vi "Convert Input Condition to Initial State.vi"(1 "Input Conditions":T2) -> (0 "Initial State":T1)   [LabVIEW 2022 SP3]
doc: "See \"Design Spreadsheet.xlsx\" for details"
uses:
  Input Conditions (cluster).ctl
  DFS Output (cluster).ctl
  Initial State (enum).ctl
panel:
  # "Development\nControls or indicators that are useful for development or testing, but which are not outputs of the VI."
  # "Input\nInputs to the VI"
  # "Output\nOutputs of the VI"
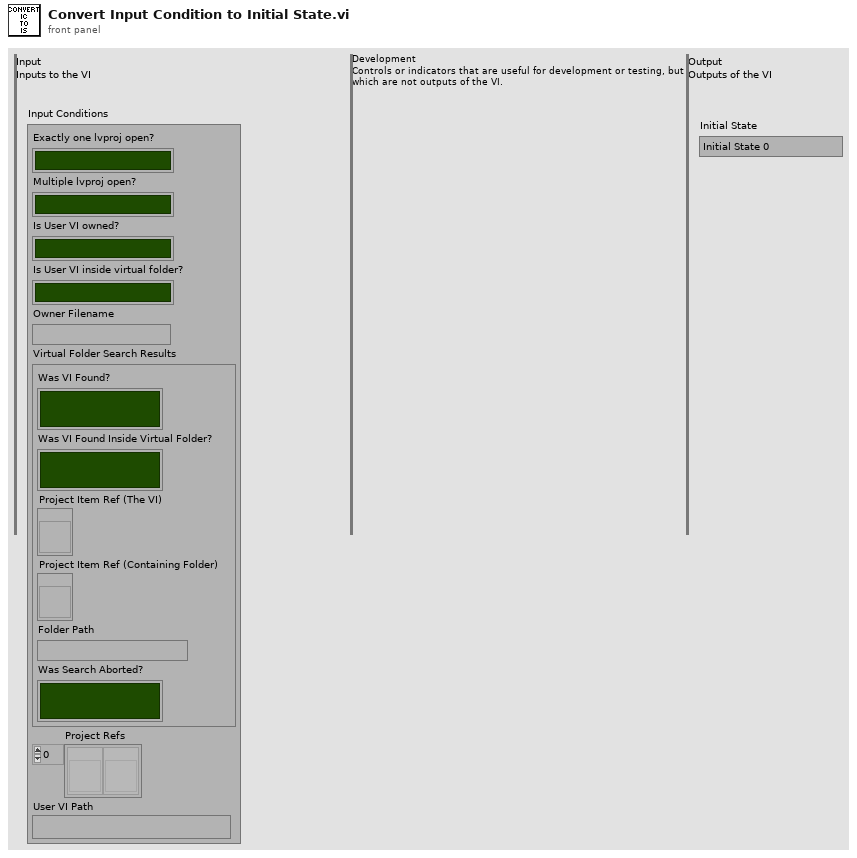
[diagram p1: front panel]
types:
  T1 = typedef "Initial State (enum).ctl" = enum16{"Initial State 0", "Initial State 1", "Initial State 2", "Initial State 3", "Initial State 4", "Initial State 5", "Initial State 6", "Initial State 7", "Initial State 8", "Initial State 9", "Initial State 10", "Initial State 11", "Initial State 12", "Initial State 13", "Initial State 14", "Initial State 15"}
  T2 = typedef "Input Conditions (cluster).ctl" = cluster{"Exactly one lvproj open?":bool, "Multiple lvproj open?":bool, "Is User VI owned?":bool, "Is User VI inside virtual folder?":bool, "Owner Filename":string, "Virtual Folder Search Results":T3, "Project Refs":refnum<vi>[], "User VI Path":path}
  T3 = typedef "DFS Output (cluster).ctl" = cluster{"Was VI Found?":bool, "Was VI Found Inside Virtual Folder?":bool, "Project Item Ref (The VI)":refnum<vi>, "Project Item Ref (Containing Folder)":refnum<vi>, "Folder Path":string, "Was Search Aborted?":bool}
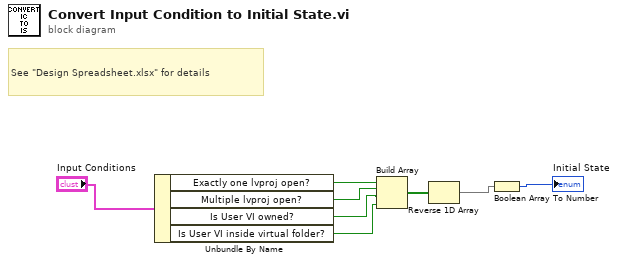
[diagram p0: block diagram]
diagram:
  # "See \"Design Spreadsheet.xlsx\" for details"
  n1 = Unbundle By Name("Input Conditions") -> ("Exactly one lvproj open?"=w7:bool, "Multiple lvproj open?"=w6:bool, "Is User VI owned?"=w5:bool, "Is User VI inside virtual folder?"=w4:bool)
  n2 = Build Array(w7, w6, w5, w4) -> (w3:bool[])
  n3 = Reverse 1D Array(array=w3) -> (reversed array=w2:bool[])
  n4 = Boolean Array To Number(Boolean array=w2) -> (number=→"Initial State":u32)
